vi "SetKeyValue_Double.vi"(6 "value":dbl, 9 "key":string, 10 "key value pairs":T1[](array[typedef])) -> (2 "key value pairs out":T1[](array[typedef]))   [LabVIEW 2017, in "PropertyHelpers.lvlib"]
doc: "Writes the double-precision, floating-point value of a particular property or key in an array of key-value pairs. This VI is useful for defining properties that the device sends to NI InsightCM Server in the form of key-value pairs within NI InsightCM message bus messages."
uses:
  <vilib>/addons/InsightCM/Utilities/PropertyHelpers/PropertyHelpers.lvlib
  <vilib>/addons/InsightCM/MessageBus/Base/controls/KeyValuePair.ctl
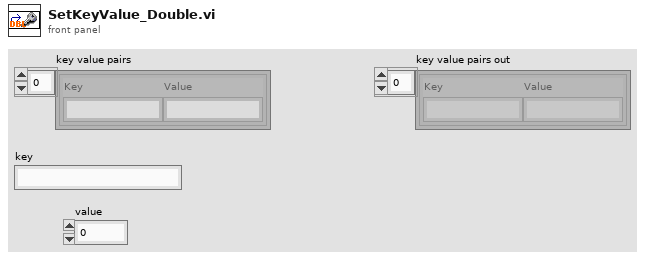
[diagram p1: front panel]
types:
  T1 = typedef "KeyValuePair.ctl" = cluster{"Key":string, "Value":string}
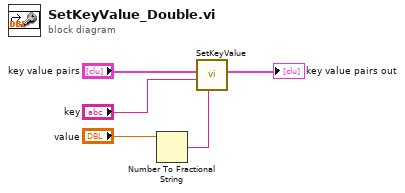
[diagram p0: block diagram]
diagram:
  n1 = Number To Fractional String(number="value") -> (F-format string=w1:string)  [unwired: 3 in]
  n2 = call <vilib>:"SetKeyValue.vi"("value"=w1, "key"="key", "key value pairs"="key value pairs") -> ("key value pairs out"=→"key value pairs out":T1[])  [unwired: 8 in]
